vi "HFRI droplet analysis v 7.0.vi"() -> ()   [LabVIEW 2021]
uses:
  <vilib>/vision/NI_Vision_Development_Module.lvlib
panel:
  out "Surface area / um2":dbl
  in  "Frame # movement bounds":cluster{i32, i32}
  out "Average speed estimate / ms-1":dbl
  out "Volume (cap) / um":dbl
  out "Contact angle / degrees":dbl
  out "Height / um":dbl
  out "Height of slices array":u8[](array[numeric])
  out "Contact radius / um":dbl
  out "Current time / s":dbl
  out "Seconds per frame":dbl
  out "Volume equivalent diameter / um":dbl
  out "Volume-equivalent radius / um":dbl
  out "Volume (slice) / um":dbl
  out "Width of slices array":u8[](array[numeric])
  out "Volume of slice":dbl[](array[numeric])
  in  "Microns / pixel":dbl=0.67264574
  out "Area of slice":dbl[](array[numeric])
  out "Contact width / um":u8
  out "Max width / um":u8
  in  "Frames per second":dbl=100000.0
  in  "Playback rate":i32=1
  in  "Resolution":cluster{"Height":i64, "Width":i64}={"Height"=128, "Width"=208}
  out "Droplet details":T1(array[cluster]) {"Aspect Ratio" format="%.2f"; "Orientation" format="%.2f"; "Area" format="%.2f"; "Object Center"."Y Centre" format="%.2f"; "Object Center"."X Centre" format="%.2f"}
  in  "Pixel Threshold":i32(slide)=151 scale=0.0..255.0
  in  "Settings":T2={"Objects"=0, "Threshold"=1, "Reject Border"=FALSE, "Fill Holes"=FALSE, "Min Object Size"=FALSE, "Min Size"=3, "Max Object Size"=FALSE, "Max Size"=100, "Show Search Area"=FALSE, "Show Center"=TRUE, "Show Bounding Box"=TRUE} {"Objects" items=["Bright Objects", "Dark Objects"]; "Threshold" min=1 max=999999999 step=1; "Max Size" min=1 max=999999999 step=1; "Min Size" min=1 max=999999999 step=1}
  out "Current Frame":i32
  out "Cropped":T3(plugin-control)
  out "File path":path caption="selected path"
  out "File name":string
  in  "stop":bool
  out "Total frames":u32
  out "Analysed Image":T3(plugin-control)
  # "High frame rate imaging droplet analysis"
  # "Input instructions"
  # "Using volume of spherical slices to calculate total volume"
  # "Calculating the contact angle of the droplet"
  # "Video Inputs"
  # "Video Data"
  # "Droplet inputs"
  # "Droplet outputs"
  # "Data files generated"
  # "Video inputs:\nSet the resolution of the actual video without saved data.\nThis will crop the superfluous data on the left hand side.\nThe actual video resolution can be found by opening the video in a media player and checking the left hand side data.\n\nSet the frame rate (the frame rate the video was captured at\nOR the frame rate at which it was saved, i.e. captured at 100,000 fps\nbut skipped every 1666 frame. Frame rate = 100,000 / 1666 = 60 fps.\n\nSet the playback rate. This is how fast the video plays below.\n\nSet the scale in microns / pixel.\n\n\nVideo data:\nThe video data fill be displayed when the program is running.\n\n\nDroplet inputs:\nSet objects to bright (the image is inverted in the image processing\nso the droplet will appear bright compared to the background).\n\nSet the threshold to 1. This is a binary image.\n\nSet various other droplet parameters depending on the video.\n\nChange the pixel threshold so the whole droplet is detected\nwhile avoiding including any background pixels.\n\nRun the program to check the pixel thresholding. Draw the ROI around the droplet area on the left hand window, taking care to accruately determine where the bottom of the droplet is (where it meets the surface) in order to cut out any of the shadow. \n\n\nDroplet outputs:\nThe droplet outputs will show the droplet:\nBounding box,\nArea,\nOrientation, \nApsect ratio, \nMax width,\nContact width,\nContact radius,\nVolume (slice),\nVolume (cap),\nHeight,\nVolume-equivalent radius,\nVolume-equivalent diameter,\nContact angle,\n\nfor each frame of the video. These values will update while the\nprogram is running\n\nTo show an estimate of the droplet speed:\nSet the frame movement bounds (first and last frame where movement is observed i.e. the frames where the free droplet is approaching the surface before impact)\n\nAn estimate of the droplet speed will be generated at the end of the program."
  # "FPS"
  # "Using the definitions for height and radius as stated here, a contact angle \ncan be calculated.\n\nUsing this equation (where length units cancel so any units are fine as long as\nthey are the same):"
  # "Two data files are generated upon running the program to completion.\n\nBoth files are created and saved in the same folder for which the selected video\nis saved (current directory).\n\n\n\nDroplet analysis_\"video file name\" saves:\n\nDroplet bounding box data\nDroplet area\nOrientation\nFrame #\nTime / s\nAspect ratio\nPixel threshold\nMax droplet width / um (widest part of the droplet, not necessarily the contact\nwidth)\nContact droplet width / um\nVolume (slices) / um3\nVolume (cap) / um3\nVolume-equivalent radius / um\nVolume-equivalent diameter / um\nHeight of spherical cap / um\nContact angle / degrees\n\n\nSpeed analysis_\"video file name\" saves:\nFrame #\nTime / s\nDistance travelled / um\nDistance travelled / m\nSpeed / ms-1"
  # "Scale"
  # "This gives a contact angle in radians.\n\nThis is converted to degrees by x 180/pi.\n\n\nThe volume of the droplet (assumed to be a spherical cap) can also be\ncalculated using these parameters.\n\nBoth the volume (slices) and this volume (cap) are calculated."
  # "The binary image is extracted as a binary arrary.\nThe sum of each row of the array is calculated. This indicates the row length.\nThe area of each row is calculated by assuming sphericity around the y axis.\n\nUsing pi*R^2 (R = half the row width) is calculate for each row.\nEach area is then converted to a volume by multiplying by the pixel height.\n\nThe sum of the volumes of these circular disks is calculated to give a total volume\nof the droplet.\n\nA volume equivalent radius is calculated from the total droplet volume."
  # "Defining the height and radius of the droplet"
  # "Calculating the speed of the droplet"
  # "The bottom of the droplet in each frame (Y bottom) is subtracted from the \nbottom of the droplet in the following frame. \n\nThis gives distance travelled per frame for each pair of frames where the droplet\nis in the shot and is moving.\n\nSpeed is calculated by dividing each distance by the time of each frame\n(1/frame rate).\n\nOften there are very few pairs of frames where the droplet is observed moving\n(i.e. where it is in flight before it impacts on the surface). Often there is only one\npair available for this speed calculation."
  # "The height and radius of \nthe dropletare defined as \nshown here.\n\nThe radius is defined as \nhalf the contact width of \nthe droplet on the surface.\n\nOften this is not the widest \npart of the droplet."
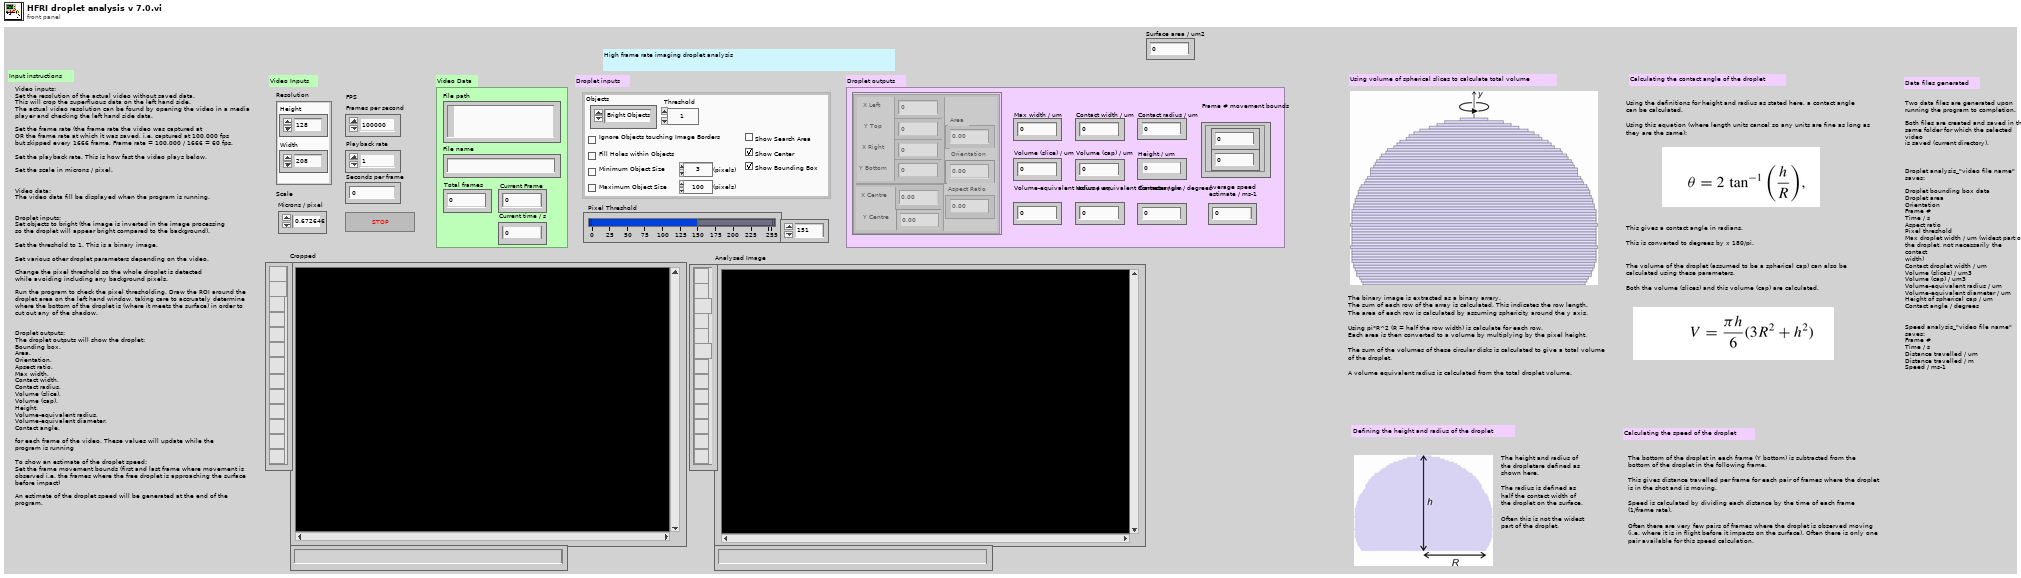
[diagram p1: front panel]
types:
  T1 = cluster{"Object Center":cluster{"X Centre":sgl, "Y Centre":sgl}, "Bounding Box":cluster{"X Left":i32, "Y Top":i32, "X Right":i32, "Y Bottom":i32}, "Area":sgl, "Orientation":sgl, "Aspect Ratio":sgl, "Nb Holes":i32}[]
  T2 = cluster{"Objects":u16, "Threshold":i32, "Reject Border":bool, "Fill Holes":bool, "Min Object Size":bool, "Min Size":i32, "Max Object Size":bool, "Max Size":i32, "Show Search Area":bool, "Show Center":bool, "Show Bounding Box":bool}
  T3 = typedef "IMAQ Image.ctl" = refnum<image>
  T4 = enum16{"open", "replace", "create", "open or create", "replace or create", "replace or create with confirmation"}
  T5 = typedef "IMAQ AVI2 Refnum.ctl" = refnum<k20>
  T6 = typedef "Image Type" = u32
  T7 = cluster{"Width":u32, "Height":u32, "Frames Per Second":u32, "Codec":string, "Has Data":bool}
  T8 = cluster{"Global Rectangle":i32[], "Contours":cluster{"Contour Type":u32, "ROI Type":u32, "Points":i32[]}[]}
  T9 = cluster{"Object Center":cluster{"X":sgl, "Y":sgl}, "Bounding Box":cluster{"X Left":i32, "Y Top":i32, "X Right":i32, "Y Bottom":i32}, "Area":sgl, "Orientation":sgl, "Aspect Ratio":sgl, "Nb Holes":i32}[]
  T10 = cluster{"Object Center":cluster{"X":sgl, "Y":sgl}, "Bounding Box":cluster{"X Left":i32, "Y Top":i32, "X Right":i32, "Y Bottom":i32}, "Area":sgl, "Orientation":sgl, "Aspect Ratio":sgl, "Nb Holes":i32}
  T11 = cluster{"X Left":i32, "Y Top":i32, "X Right":i32, "Y Bottom":i32}
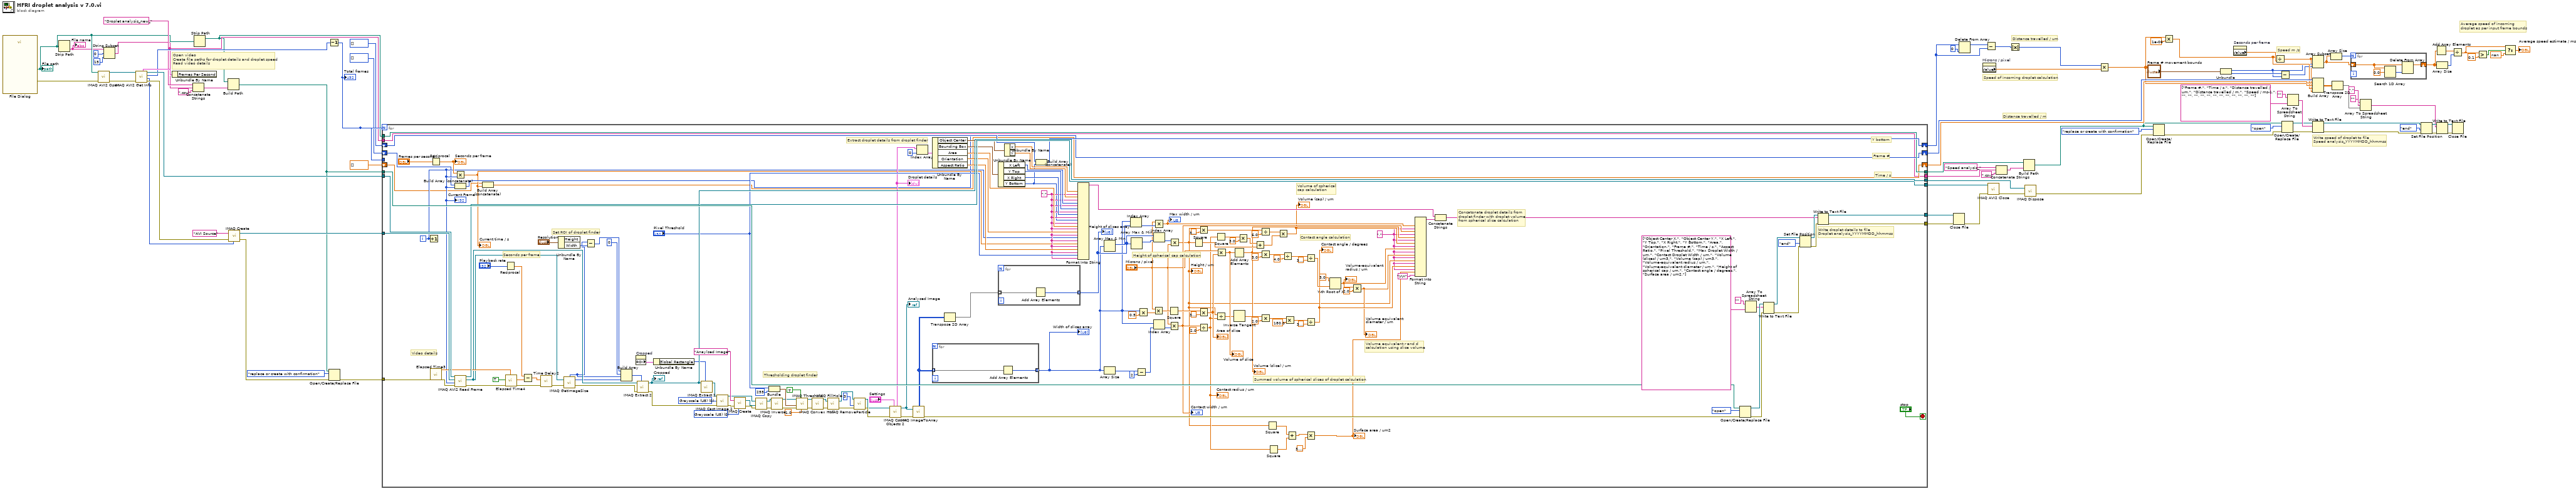
[diagram p0: block diagram]
diagram:
  # "Average speed of incoming\ndroplet as per input frame bounds"
  # "Open video\nCreate file paths for droplet details and droplet speed\nRead video details"
  # "Write speed of droplet to file\nSpeed analysis_YYYYMMDD_hhmmss"
  # "Speed of incoming droplet calculation"
  # "Speed m /s"
  # "Distance travelled / m"
  # "Distance travelled / um"
  n1 = call "File Dialog"() -> ("selected path"=w61:path, "error out"=w76:errorcluster)  [unwired: 12 in, 2 out]
  "File path" <- w61
  n2 = Strip Path(path=w61) -> (name=w60:string)  [unwired: 1 out]
  "File name" <- w60
  n3 = call "IMAQ AVI2 Open"("error in (no error)"=w76, "AVI File Path"=w61) -> ("error out"=w87:errorcluster, "AVI Refnum"=w86:T5)  [unwired: 8 in]
  n4 = String Subset(string=w60, offset (0)=0, length (rest)=15 ("length (rest)")) -> (substring=w23:string)
  n5 = call "IMAQ AVI2 Get Info"("error in (no error)"=w87, "AVI Refnum"=w86) -> ("error out"=w84:errorcluster, "Image Type"=w83:T6, "Number of Frames"=w73:u32, "AVI Refnum (duplicate)"=w81:T5, "Frame Data"=w85:T7)  [unwired: 5 in]
  n6 = Unbundle By Name(w85) -> ()  [unwired: 1 out]
  n7 = Concatenate Strings("Droplet analysis_new_" ("time format string (%c)"), w23, ".csv") -> (w69:string)
  n8 = Strip Path(path=w61) -> (stripped path=w22:path)  [unwired: 1 out]
  n9 = Build Path(base path=w22, name or relative path=w69) -> (appended path=w65:path)
  n10 = call "IMAQ Create"("Image Name"="AVI Source", "Image Type"=w83, "error in (no error)"=w84) -> ("New Image"=w80:T3, "error out"=w64:errorcluster)  [unwired: 2 in]
  n11 = Decrement(x=w73) -> (x-1=w71:u32)
  "Total frames" <- w71
  n12 = Open/Create/Replace File(file path (use dialog)=w65, error in=w64, operation (0:open)=T4."replace or create with confirmation") -> (error out=w63:errorcluster)  [unwired: 3 in, 2 out]
  n13 = for {
    N: w71 -> [_]
    tunnel: w81 -> [w248]
    tunnel: w80 -> [w247]
    tunnel: w63 -> [w246]
    tunnel: [w244] -> w79
    tunnel: [w245] -> w78
    tunnel: w71 -> [_]
    tunnel: [w243] -> w75
    tunnel: [w242] -> w74
    tunnel: w65 -> [w249]
    shift-right: [w140] -> w50
    shift-left: i32[] [] -> [w139]
    tunnel: w22 -> [w138]
    tunnel: [w138] -> w19
    shift-right: [w136] -> w49
    shift-left: i32[] [] -> [w135]
    shift-right: [w133] -> w48
    shift-left: dbl[] [] -> [w132]
    tunnel: w23 -> [w131]
    tunnel: [w131] -> w21
    i -> [w137]
    stop <- "stop" stop-if-true
    w147 = ","
    w89 = ","
    w231 = T6 0 items=["Grayscale (U8)", "Grayscale (I16)", "Grayscale (SGL)", "Complex (CSG)", "RGB (U32)", "HSL (U32)", "RGB (U64)", "Grayscale (U16)"] ("Image Type")
    w232 = T6 0 items=["Grayscale (U8)", "Grayscale (I16)", "Grayscale (SGL)", "Complex (CSG)", "RGB (U32)", "HSL (U32)", "RGB (U64)", "Grayscale (U16)"] ("Image Type")
    # "Volume equivalent r and d \ncalculation using slice volume"
    # "Volume of spherical\ncap calculation"
    # "Contact angle calculation"
    # "Height of spherical cap calculation"
    # "Concatonate droplet details from\ndroplet finder with droplet volume\nfrom spherical slice calculation"
    # "Extract droplet details from droplet finder"
    # "Video details"
    # "Thresholding droplet finder"
    # "Set ROI of droplet finder"
    # "Write droplet details to file\nDroplet analysis_YYYYMMDD_hhmmss"
    # "Summed volume of spherical slices of droplet calculation"
    # "Time / s"
    # "Frame #"
    # "Y bottom"
    # "Seconds per frame"
    n14 = Increment(x=w137) -> ()  [unwired: 1 out]
    n15 = Reciprocal(x="Frames per second") -> (1/x=w150:dbl)
    "Seconds per frame" <- w150
    n16 = call "Elapsed Time3"("error in (no error)"=w246) -> ("Present (s)"=w234:dbl, "error out"=w239:errorcluster)  [unwired: 11 in, 6 out]
    n17 = Multiply(x=w150, y=w137) -> (x*y=w134:dbl)
    "Current time / s" <- w134
    n18 = Build Array (concatenate)(w135, w137) -> (w136:i32[])
    n19 = call "IMAQ AVI2 Read Frame"("error in (no error)"=w239, "Frame Number"=w137, "Image"=w247, "AVI Refnum"=w248) -> ("error out"=w200:errorcluster, "Image Out"=w194:T3, "AVI Refnum (duplicate)"=w244:T5)  [unwired: 5 in]
    n20 = Build Array (concatenate)(w132, w134) -> (w133:dbl[])
    n21 = Reciprocal(x="Playback rate") -> (1/x=w241:dbl)
    n22 = call "Elapsed Time4"("Reset"=TRUE, "error in (no error)"=w200, "Set Start Time (s)"=w234) -> ("Elapsed Time (s)"=w237:dbl, "error out"=w235:errorcluster)  [unwired: 9 in, 6 out]
    n23 = Subtract(x=w241, y=w237) -> (x-y=w236:dbl)
    n24 = call "Time Delay2"("error in (no error)"=w235, "Delay Time (s)"=w236) -> ("error out"=w197:errorcluster)  [unwired: 9 in]
    n25 = Unbundle By Name("Resolution") -> ("Width"=w190:i64)  [unwired: 1 out]
    n26 = call "IMAQ GetImageSize"("Image"=w194, "error in (no error)"=w197) -> ("Y Resolution"=w188:i32, "X Resolution"=w189:i32, "error out"=w196:errorcluster)  [unwired: 2 in]
    n27 = Subtract(x=w189, y=w190) -> (x-y=w193:i64)
    n28 = Build Array(w193, i64 0 ("element"), w189, w188) -> (w191:i64[])
    n29 = property on="Cropped" class="ImageControl"() -> ("ROI"=w186:T8)  [unwired: 2 in, 2 out]
    n30 = call "IMAQ Extract 2"("Optional Rectangle"=w191, "error in (no error)"=w196, "Image Src"=w194) -> ("error out"=w195:errorcluster, "Image Dst Out"=w245:T3)  [unwired: 7 in]
    "Cropped" <- w245
    n31 = Unbundle By Name(w186) -> ("Global Rectangle"=w185:i32[])
    n32 = call "IMAQ Extract 2"("Optional Rectangle"=w185, "Image Src"=w245) -> ("Image Dst Out"=w187:T3)  [unwired: 8 in, 1 out]
    n33 = call "IMAQ Cast Image 2"("Image Src"=w187, "Image Type"=w232, "error in (no error)"=w195) -> ("Image Dst Out"=w227:T3, "error out"=w233:errorcluster)  [unwired: 11 in]
    n34 = call "IMAQ Create"("Image Name"="Anaylsed Image", "Image Type"=w231, "error in (no error)"=w233) -> ("New Image"=w228:T3, "error out"=w229:errorcluster)  [unwired: 2 in]
    n35 = call "IMAQ Copy"("error in (no error)"=w229, "Image Dst"=w228, "Image Src"=w227) -> ("error out"=w226:errorcluster, "Image Dst Out"=w204:T3)  [unwired: 3 in]
    n36 = Bundle("Pixel Threshold"="Pixel Threshold", 255) -> (w223:cluster{"Pixel Threshold":i32, i32})  [unwired: 1 in]
    n37 = call "IMAQ Inverse"("error in (no error)"=w226, "Image Src"=w204) -> ("error out"=w225:errorcluster, "Image Dst Out"=w206:T3)  [unwired: 8 in]
    n38 = call "IMAQ Threshold"("Replace Value"=sgl 1.0, "Keep/Replace Value (Replace)"=TRUE, "error in (no error)"=w225, "Range"=w223, "Image Src"=w206) -> ("error out"=w220:errorcluster, "Image Dst Out"=w203:T3)  [unwired: 5 in]
    n39 = call "IMAQ Convex Hull"("error in (no error)"=w220, "Image Src"=w203) -> ("error out"=w219:errorcluster, "Image Dst Out"=w201:T3)  [unwired: 8 in]
    n40 = call "IMAQ FillHole"("error in (no error)"=w219, "Image Src"=w201) -> ("error out"=w183:errorcluster, "Image Dst Out"=w184:T3)  [unwired: 4 in]
    n41 = call "IMAQ RemoveParticle"("error in (no error)"=w183, "Number of Erosion"=3, "Image Src"=w184) -> ("error out"=w218:errorcluster, "Image Dst Out"=w202:T3)  [unwired: 7 in]
    n42 = call "IMAQ Count Objects 2"("Settings"="Settings", "error in (no error)"=w218, "Image"=w202) -> ("error out"=w180:errorcluster, "Image Out"=w181:T3, "Objects"=w146:T9)  [unwired: 4 in, 2 out]
    "Droplet details" <- w146
    "Analysed Image" <- w181
    n43 = call "IMAQ ImageToArray"("error in (no error)"=w180, "Image"=w181) -> ("error out"=w199:errorcluster, "Image Pixels (U8)"=w128:u8[][])  [unwired: 2 in, 3 out]
    n44 = Index Array(array=w146, index=0) -> (element=w144:T10)
    n45 = Unbundle By Name(w144) -> ("Object Center"=w151:cluster{"X":sgl, "Y":sgl}, "Bounding Box"=w154:T11, "Area"=w158:sgl, "Orientation"=w159:sgl, "Aspect Ratio"=w148:sgl)
    n46 = for {
      tunnel: w128 -> [w254] mode=indexing
      tunnel: [w253] -> w122 mode=indexing
      n47 = Add Array Elements(numeric array=w254) -> (sum=w253:u8)
    }
    "Width of slices array" <- w122
    n48 = Transpose 2D Array(2D array=w128) -> (transposed array=w127:u8[][])
    n49 = Unbundle By Name(w154) -> ("X Left"=w155:i32, "Y Top"=w156:i32, "X Right"=w157:i32, "Y Bottom"=w141:i32)
    n50 = for {
      tunnel: [w252] -> w125 mode=indexing
      tunnel: w127 -> [w251] mode=indexing
      n51 = Add Array Elements(numeric array=w251) -> (sum=w252:u8)
    }
    "Height of slices array" <- w125
    n52 = Unbundle By Name(w151) -> ("X"=w152:sgl, "Y"=w153:sgl)
    n53 = Build Array (concatenate)(w139, w141) -> (w140:i32[])
    n54 = Format Into String(w152, w147, w153, w147, w155, w147, w156, w147, w157, w147, w141, w147, w158, w147, w159, w147, w137, w147, w134, w147, w148, w147, "Pixel Threshold", w147) -> (resulting string=w143:string)  [unwired: 3 in, 1 out]
    n55 = Array Max & Min(array=w122) -> (max index (indices)=w179:i32)  [unwired: 3 out]
    n56 = Array Size(array=w122) -> (size(s)=w120:i32)
    n57 = Index Array(array=w122, index=w179) -> (element=w164:u8)
    n58 = Array Max & Min(array=w125) -> (max index (indices)=w126:i32)  [unwired: 3 out]
    n59 = Subtract(x=w120, y=2) -> (x-y=w121:i32)
    n60 = Multiply(x=w122, y=0.5) -> (x*y=w173:dbl[])
    n61 = Multiply(x="Microns / pixel", y=w173) -> (x*y=w175:dbl[])
    n62 = Multiply(x="Microns / pixel", y=w164) -> (x*y=w160:dbl)
    "Max width / um" <- w160
    n63 = Index Array(array=w125, index=w126) -> (element=w124:u8)
    n64 = Index Array(array=w122, index=w121) -> (element=w118:u8)
    n65 = Square(x=w175) -> (x^2=w178:dbl[])
    n66 = Multiply(x="Microns / pixel", y=w118) -> (x*y=w130:dbl)
    "Contact width / um" <- w130
    n67 = Multiply(x=w124, y="Microns / pixel") -> (x*y=w93:dbl)
    "Height / um" <- w93
    n68 = Square(x=w93) -> (x^2=w103:dbl)
    n69 = Multiply(x=w93, y=3.141592653589793) -> (x*y=w106:dbl)
    n70 = Multiply(x=w178, y=3.141592653589793) -> (x*y=w176:dbl[])
    "Area of slice" <- w176
    n71 = Divide(x=w130, y=2.0) -> (x/y=w96:dbl)
    "Contact radius / um" <- w96
    n72 = Square(x=w96) -> (x^2=w110:dbl)
    n73 = Divide(x=w93, y=w96) -> (x/y=w117:dbl)
    n74 = Multiply(x="Microns / pixel", y=w176) -> (x*y=w172:dbl[])
    "Volume of slice" <- w172
    n75 = Add Array Elements(numeric array=w172) -> (sum=w101:dbl)
    "Volume (slice) / um" <- w101
    n76 = Inverse Tangent(1:w117) -> (0:w116:dbl)
    n77 = Multiply(x=w110, y=3.0) -> (x*y=w108:dbl)
    n78 = Add(x=w108, y=w103) -> (x+y=w102:dbl)
    n79 = Divide(x=w106, y=6.0) -> (x/y=w104:dbl)
    n80 = Multiply(x=w101, y=3.0) -> (x*y=w170:dbl)
    n81 = Multiply(x=w116, y=2.0) -> (x*y=w114:dbl)
    n82 = Square(x=w93) -> (x^2=w94:dbl)
    n83 = Square(x=w96) -> (x^2=w95:dbl)
    n84 = Multiply(x=w104, y=w102) -> (x*y=w97:dbl)
    "Volume (cap) / um" <- w97
    n85 = Divide(x=w170, y=4.0) -> (x/y=w168:dbl)
    n86 = Multiply(x=w114, y=180.0) -> (x*y=w112:dbl)
    n87 = Add(x=w94, y=w95) -> (x+y=w92:dbl)
    n88 = Divide(x=w168, y=3.141592653589793) -> (x/y=w166:dbl)
    n89 = Divide(x=w112, y=3.141592653589793) -> (x/y=w100:dbl)
    "Contact angle / degrees" <- w100
    n90 = Multiply(x=w92, y=3.141592653589793) -> (x*y=w88:dbl)
    "Surface area / um2" <- w88
    n91 = Y-th Root of X(1:w166, 2:3.0 ("y")) -> (0:w98:dbl)
    "Volume-equivalent radius / um" <- w98
    n92 = Multiply(x=w98, y=2.0) -> (x*y=w99:dbl)
    "Volume equivalent diameter / um" <- w99
    n93 = Format Into String(w160, w89, w130, w89, w101, w89, w97, w89, w98, w89, w99, w89, w93, w89, w100, w89, w88, "\r\n") -> (resulting string=w142:string)  [unwired: 3 in, 1 out]
    n94 = Concatenate Strings(w143, w142) -> (w161:string)
    n95 = Open/Create/Replace File(file path (use dialog)=w249, error in=w199, operation (0:open)=T4."open") -> (refnum out=w212:refnum<file>, error out=w213:errorcluster)  [unwired: 3 in, 1 out]
    n96 = Array To Spreadsheet String(array=string[] ["Object Center X,", "Object Center Y,", "X Left,", "Y Top,", "X Right,", "Y Bottom,", "Area,", "Orientation,", "Frame #,", "Time / s,", "Aspect Ratio,", "Pixel Threshold,", "Max Droplet Width / um,", "Contact Droplet Width / um,", "Volume (slices) / um3,", "Volume (cap) / um3,", "Volume-equivalent radius / um,", "Volume-equivalent diameter / um,", "Height of spherical cap / um,", "Contact angle / degrees,", "Surface area / um2,"], 3:"" ("format string")) -> (spreadsheet string=w210:string)  [unwired: 1 in]
    n97 = Write to Text File(file (use dialog)=w212, text=w210, error in=w213) -> (refnum out=w214:refnum<file>, error out=w215:errorcluster)  [unwired: 1 in, 1 out]
    n98 = Set File Position(refnum=w214, from (0:start)=enum16{"start", "end", "current"}."end", error in=w215) -> (refnum out=w207:refnum<file>, error out=w208:errorcluster)  [unwired: 1 in]
    n99 = Write to Text File(file (use dialog)=w207, text=w161, error in=w208) -> (refnum out=w243:refnum<file>, error out=w242:errorcluster)  [unwired: 1 in, 1 out]
    "Current Frame" <- w137
  }
  n100 = Close File(refnum=w75, error in=w74) -> (error out=w72:errorcluster)  [unwired: 1 out]
  n101 = Delete From Array(array=w50, index=0) -> (array with subset deleted=w58:i32[])  [unwired: 1 in, 1 out]
  n102 = property on="Microns / pixel" class="DigNum (strict)"() -> ("Value"=w57:dbl)  [unwired: 2 in, 2 out]
  n103 = Subtract(x=w58, y=w50) -> (x-y=w29:i32[])
  n104 = call "IMAQ AVI2 Close"("error in (no error)"=w72, "AVI Refnum"=w79) -> ("error out"=w77:errorcluster)  [unwired: 9 in]
  n105 = Concatenate Strings("Speed analysis_" ("time format string (%c)"), w21, ".csv") -> (w54:string)
  n106 = Absolute Value(x=w29) -> (abs(x)=w28:i32[])
  n107 = Build Path(base path=w19, name or relative path=w54) -> (appended path=w20:path)
  n108 = call "IMAQ Dispose"("Image"=w78, "error in (no error)"=w77) -> ("error out"=w51:errorcluster)  [unwired: 4 in]
  n109 = Multiply(x=w28, y=w57) -> (x*y=w47:dbl[])
  n110 = Open/Create/Replace File(file path (use dialog)=w20, error in=w51, operation (0:open)=T4."replace or create with confirmation") -> (error out=w27:errorcluster)  [unwired: 3 in, 2 out]
  n111 = Multiply(x=w47, y=1e-06) -> (x*y=w46:dbl[])
  n112 = Unbundle("Frame # movement bounds") -> (w8:i32, w10:i32)
  n113 = property on="Seconds per frame" class="DigNum (strict)"() -> ("Value"=w55:dbl)  [unwired: 2 in, 2 out]
  n114 = Divide(x=w46, y=w55) -> (x/y=w7:dbl[])
  n115 = Subtract(x=w10, y=w8) -> (x-y=w9:i32)
  n116 = Open/Create/Replace File(file path (use dialog)=w20, error in=w27, operation (0:open)=T4."open") -> (refnum out=w25:refnum<file>, error out=w26:errorcluster)  [unwired: 3 in, 1 out]
  n117 = Array To Spreadsheet String(array=string[] ["Frame #,", "Time / s,", "Distance travelled / um,", "Distance travelled / m,", "Speed / ms-1,", "", "", "", "", "", "", "", "", "", "", "", ""], 3:"" ("format string")) -> (spreadsheet string=w31:string)  [unwired: 1 in]
  n118 = Array Subset(array=w7, index=w8, length=w9) -> (w6:dbl[])
  n119 = Build Array(w49, w48, w47, w46, w7) -> (w45:dbl[][])
  n120 = Write to Text File(file (use dialog)=w25, text=w31, error in=w26) -> (refnum out=w42:refnum<file>, error out=w43:errorcluster)  [unwired: 1 in, 1 out]
  n121 = Array Size(array=w6) -> (size(s)=w15:i32)
  n122 = Transpose 2D Array(2D array=w45) -> (transposed array=w34:dbl[][])
  n123 = for {
    N: w15 -> [_]
    shift-right: [w256] -> w13
    shift-left: w6 -> [w255]
    n124 = Search 1D Array(1D array=w255, element=0.0) -> (index of element=w257:i32)  [unwired: 1 in]
    n125 = Delete From Array(array=w255, index=w257) -> (array with subset deleted=w256:dbl[])  [unwired: 1 in, 1 out]
  }
  n126 = Array To Spreadsheet String(delimiter (Tab)="," ("format string"), array=w34, 3:"" ("format string")) -> (spreadsheet string=w32:string)
  n127 = Set File Position(refnum=w42, from (0:start)=enum16{"start", "end", "current"}."end", error in=w43) -> (refnum out=w39:refnum<file>, error out=w40:errorcluster)  [unwired: 1 in]
  n128 = Add Array Elements(numeric array=w13) -> (sum=w14:dbl)
  n129 = Array Size(array=w13) -> (size(s)=w12:i32)
  n130 = Write to Text File(file (use dialog)=w39, text=w32, error in=w40) -> (refnum out=w37:refnum<file>, error out=w38:errorcluster)  [unwired: 1 in, 1 out]
  n131 = Divide(x=w14, y=w12) -> (x/y=w4:dbl)
  n132 = Close File(refnum=w37, error in=w38) -> ()  [unwired: 2 out]
  n133 = Greater?(x=w4, y=0.1) -> (0:w2:bool)
  n134 = Select(t=w4, s=w2, f=nan) -> (s? t:f=→"Average speed estimate / ms-1":dbl)
